vi "Convert to Eng, P only.vi"(0 "Pmin (Pa)":sgl format="%#_13g", 1 "OutputMin (counts)":sgl format="%#_13g", 2 "Poffset (Pa)":sgl format="%#_13g", 3 "(Pmax - Pmin) / (OutputMax - OutputMin) (Pa/count)":sgl format="%#_13g", 4 "P word":string) -> (5 "P (Pa)":sgl, 6 "Status bits":u8)   [LabVIEW 2015]
panel:
  # "0: valid data\n1: cmd mode\n2: stale data\n3: diag mode"
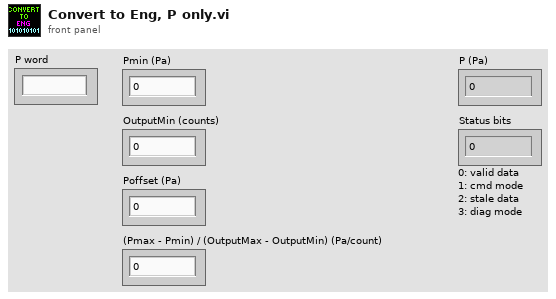
[diagram p1: front panel]
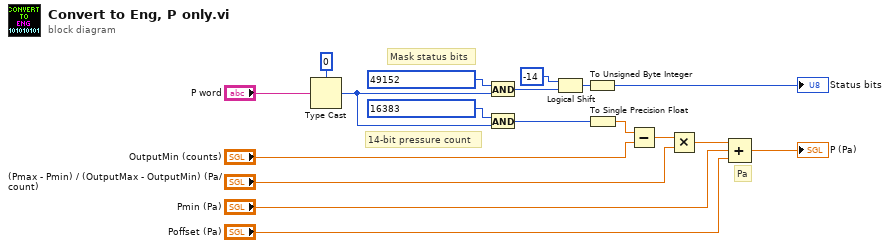
[diagram p0: block diagram]
diagram:
  # "Pa"
  # "14-bit pressure count"
  # "Mask status bits"
  n1 = Type Cast(type=u16 0, x="P word") -> (*(type *) &x=w1:u16)
  n2 = And(x=u16 49152, y=w1) -> (x .and. y?=w8:u16)
  n3 = And(x=u16 16383, y=w1) -> (x .and. y?=w14:u16)
  n4 = Logical Shift(y=i16 -14, x=w8) -> (x << y=w10:u16)
  n5 = To Unsigned Byte Integer(number=w10) -> (unsigned 8bit integer=→"Status bits":u8)
  n6 = To Single Precision Float(number=w14) -> (single precision float=w15:sgl)
  n7 = Subtract(x=w15, y="OutputMin (counts)") -> (x-y=w16:sgl)
  n8 = Multiply(x=w16, y="(Pmax - Pmin) / (OutputMax - OutputMin) (Pa/count)") -> (x*y=w4:sgl)
  n9 = Compound Arithmetic op=ADD(w4, "Pmin (Pa)", "Poffset (Pa)") -> (→"P (Pa)":sgl)
